vi "Point_Write_string.vi"(6 "Time Stamp":timestamp, 7 "Auto Create?":bool=TRUE, 8 "Error In":errorcluster, 9 "Value":string, 10 "Tag":string, 11 "Map":T1) -> (0 "Error Out":errorcluster, 3 "Map Out":T1)   [LabVIEW 2017, in "PointValueMap.lvlib"]
doc: "Sets the value of a map point. If the point does not exist, you can optionally create the point. Wire data to the <B>Value</B> input to determine the polymorphic instance to use."
uses:
  <vilib>/addons/PointValueMap/PointValueMap.lvlib
  <vilib>/addons/PointValueMap/controls/PointMap.ctl
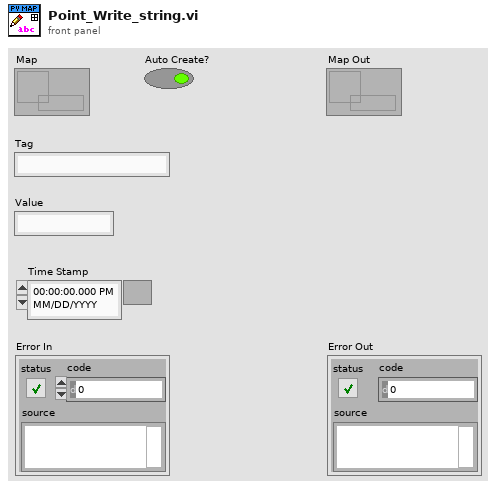
[diagram p1: front panel]
types:
  T1 = typedef "PointValueMap.lvlib/PointMap.ctl" = refnum<data-value>
  T2 = typedef "PointValueMap.lvlib/Point.ctl" = cluster{"Datatype":T3, "Timestamp":timestamp, "Value":variant, "Valid":bool}
  T3 = typedef "PointValueMap.lvlib/DataTypes.ctl" = enum16{"single", "double", "i32", "string", "variant"}
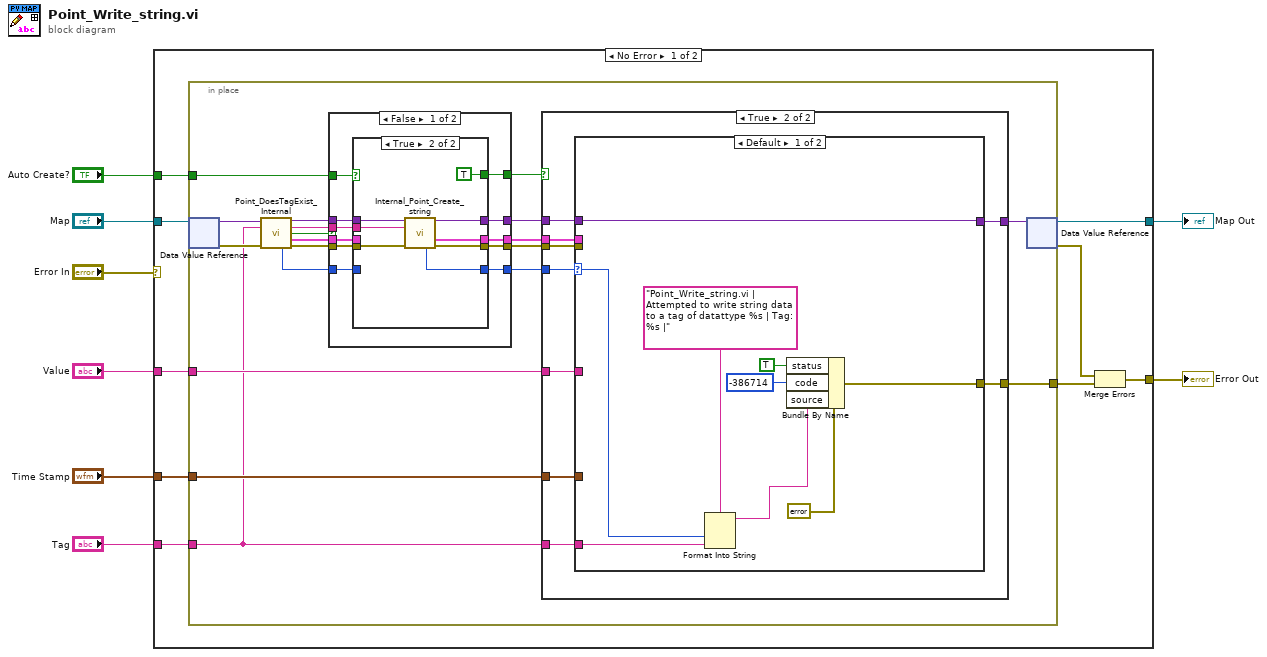
[diagram p0: block diagram]
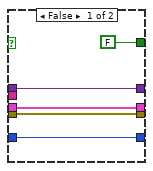
[diagram p2: hidden frame]
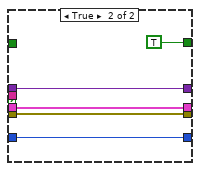
[diagram p3: hidden frame]
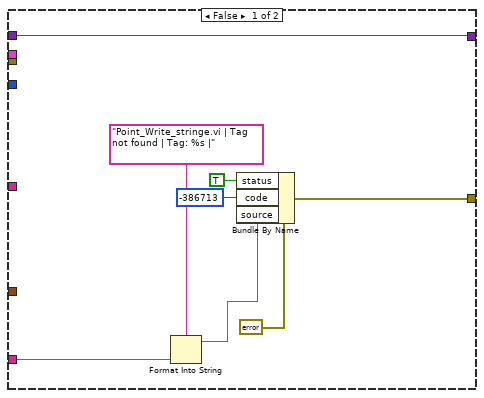
[diagram p4: hidden frame]
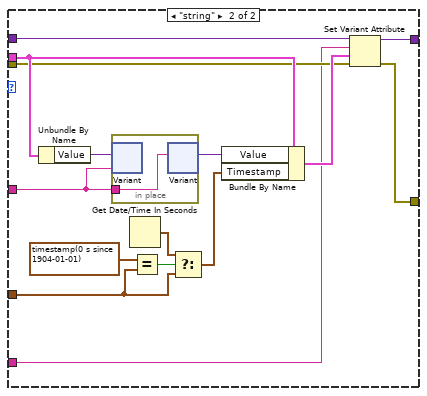
[diagram p5: hidden frame]
diagram:
  n1 = case shown="No Error" "Error In" {
    selector: "Error In" -> [_ w109]
    tunnel: "Map" -> [w17 w108]
    tunnel: "Tag" -> [w16 _]
    tunnel: [w13 w109] -> w7
    tunnel: "Value" -> [w12 _]
    tunnel: "Time Stamp" -> [w11 _]
    tunnel: [w10 w108] -> w3
    tunnel: "Auto Create?" -> [w9 _]
    frame No Error {
      n2 = in-place {
        in-place-border: w16 -> [w23]
        in-place-border: [w35] -> w14
        in-place-border: w12 -> [w34]
        in-place-border: w11 -> [w33]
        in-place-border: w9 -> [w30]
        n3 = in-place-dvr #1(w17) -> (w32:variant, w31:errorcluster)
        n4 = call <vilib>:"Point_DoesTagExist_Internal.vi"("Map"=w32, "Tag"=w23, "Error In"=w31) -> ("Map Out"=w27:variant, "Tag Out"=w18:string, "Tag Exists"=w29:bool, "Point"=w20:T2, "Datatype"=w21:T3, "Error Out"=w25:errorcluster)  [unwired: 7 in]
        n5 = case shown="False" w29 {
          tunnel: w30 -> [w47 _]
          tunnel: [w45 w65] -> w28
          tunnel: w27 -> [w44 w65]
          tunnel: [w43 w64] -> w26
          tunnel: w25 -> [w42 w64]
          tunnel: [w46 TRUE] -> w24
          tunnel: [w41 w62] -> w22
          tunnel: w21 -> [w40 w62]
          tunnel: w20 -> [w39 w61]
          tunnel: [w38 w61] -> w19
          tunnel: w18 -> [w37 _]
          frame False {
            n6 = case shown="True" w47 {
              tunnel: [FALSE TRUE] -> w46
              tunnel: [w51 w57] -> w45
              tunnel: w44 -> [w51 w60]
              tunnel: [w50 w58] -> w43
              tunnel: w42 -> [w50 w59]
              tunnel: [w49 w55] -> w41
              tunnel: w40 -> [w49 _]
              tunnel: w39 -> [w48 _]
              tunnel: [w48 w54] -> w38
              tunnel: w37 -> [_ w53]
              frame False {
              }
              frame True {
                n7 = call <vilib>:"Internal_Point_Create_string.vi"("Internal Map (variant)"=w60, "Tag Name"=w53, "error in (no error)"=w59) -> ("Internal Map Out (variant)"=w57:variant, "Point"=w54:T2, "Datatype"=w55:T3, "error out"=w58:errorcluster)  [unwired: 8 in, 1 out]
              }
            }
          }
          frame True {
          }
        }
        n8 = case shown="True" w24 {
          tunnel: [w66 w82] -> w36
          tunnel: [w68 w81] -> w35
          tunnel: w34 -> [_ w80]
          tunnel: w33 -> [_ w79]
          tunnel: w26 -> [_ w78]
          tunnel: w28 -> [w66 w77]
          tunnel: w22 -> [_ w76]
          tunnel: w23 -> [w67 w75]
          tunnel: w19 -> [_ w74]
          frame False {
            n9 = Format Into String(format string="Point_Write_stringe.vi | Tag not found | Tag: %s |" ("source"), w67) -> (resulting string=w70:string)  [unwired: 2 in, 1 out]
            n10 = Bundle By Name(cluster=errorcluster {"status"=FALSE, "code"=0, "source"=""} ("Error Out"), "status"=TRUE, "code"=-386713, "source"=w70) -> (w68:errorcluster)
          }
          frame True {
            n11 = case shown="Default" w76 {
              selector: w76 -> [w83 _]
              tunnel: w77 -> [w84 w99]
              tunnel: w78 -> [_ w100]
              tunnel: [w84 w103] -> w82
              tunnel: [w87 w102] -> w81
              tunnel: w80 -> [_ w97]
              tunnel: w79 -> [_ w92]
              tunnel: w75 -> [w85 w98]
              tunnel: w74 -> [_ w104]
              frame Default {
                n12 = Format Into String(format string="Point_Write_string.vi | Attempted to write string data to a tag of datattype %s | Tag: %s |" ("source"), w83, w85) -> (resulting string=w88:string)  [unwired: 2 in, 1 out]
                n13 = Bundle By Name(cluster=errorcluster {"status"=FALSE, "code"=0, "source"=""} ("Error Out"), "status"=TRUE, "code"=-386714, "source"=w88) -> (w87:errorcluster)
              }
              frame "string" {
                n14 = Unbundle By Name(w104) -> ("Value"=w106:variant)
                n15 = in-place {
                  in-place-border: w97 -> [w107]
                  n16 = in-place-variant #2(w106, w97) -> ()  [unwired: 2 out]
                  n17 = in-place-variant #2(w107) -> (w105:variant)  [unwired: 1 out]
                }
                n18 = Get Date/Time In Seconds() -> (seconds since 1Jan1904=w94:timestamp)
                n19 = Equal?(x=timestamp(0 s since 1904-01-01) ("Timestamp"), y=w92) -> (x = y?=w96:bool)
                n20 = Select(t=w94, s=w96, f=w92) -> (s? t:f=w93:timestamp)
                n21 = Bundle By Name(cluster=w104, "Value"=w105, "Timestamp"=w93) -> (w101:T2)
                n22 = Set Variant Attribute(Variant=w99, name=w98, value=w101, error in=w100) -> (Variant out=w103:variant, error out=w102:errorcluster)  [unwired: 1 out]
              }
            }
          }
        }
        n23 = in-place-dvr #1(w36) -> (w10:T1, w15:errorcluster)
      }
      n24 = Merge Errors(w15, w14) -> (w13:errorcluster)
    }
    frame Error {
    }
  }
  "Error Out" <- w7
  "Map Out" <- w3
